vi "sqiggle_write_n.vi"(7 "I2C interface":T1, 8 "error in":errorcluster, 10 "Axis num":i32, 11 "Pulse count":i16) -> (0 "error out":errorcluster)   [LabVIEW 2013]
uses:
  i2c_interface.ctl
  fpga_reference.ctl
  Common/demux_command.ctl
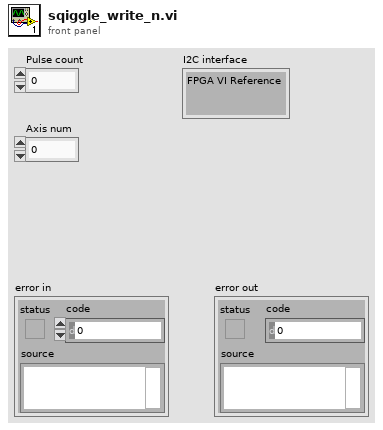
[diagram p1: front panel]
types:
  T1 = typedef "i2c_interface.ctl" = cluster{"FPGA VI Reference":T2}
  T2 = typedef "fpga_reference.ctl" = refnum<k20>
  T3 = typedef "demux_command.ctl" = enum8{"bus_0", "bus_1", "bus_2", "invalid_3", "invalid_4", "drain_fifo", "wait_hard_trigger", "wait_soft_trigger", "trigger_enable"}
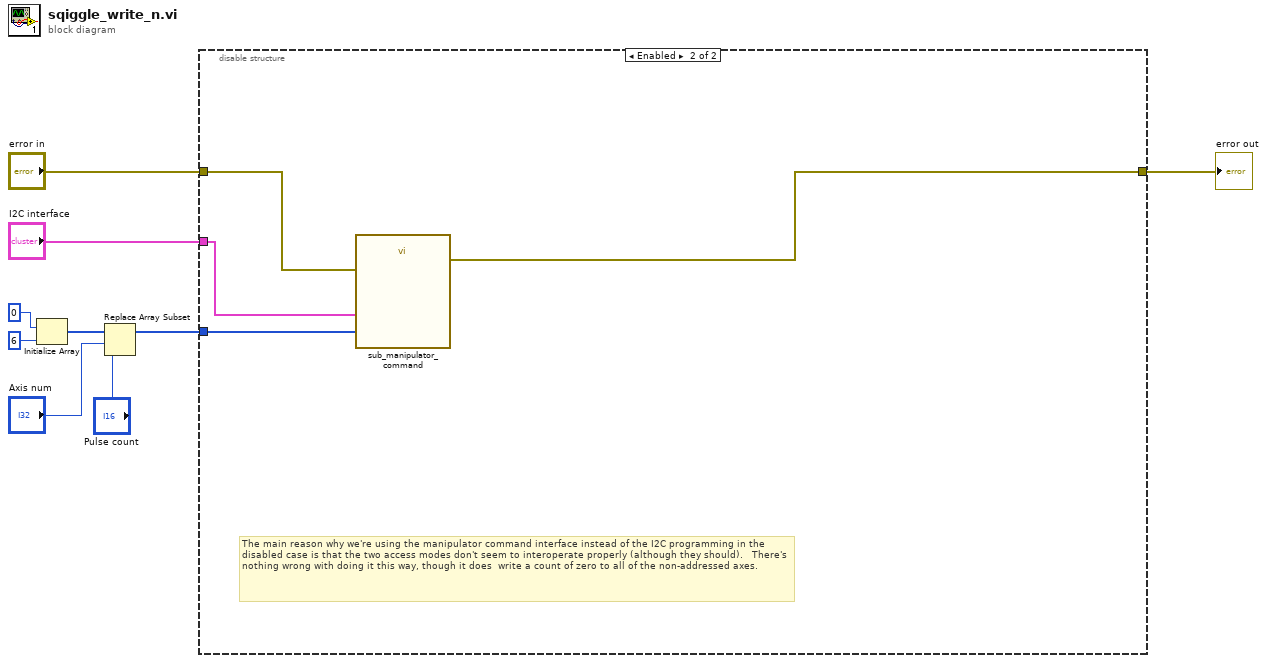
[diagram p0: block diagram]
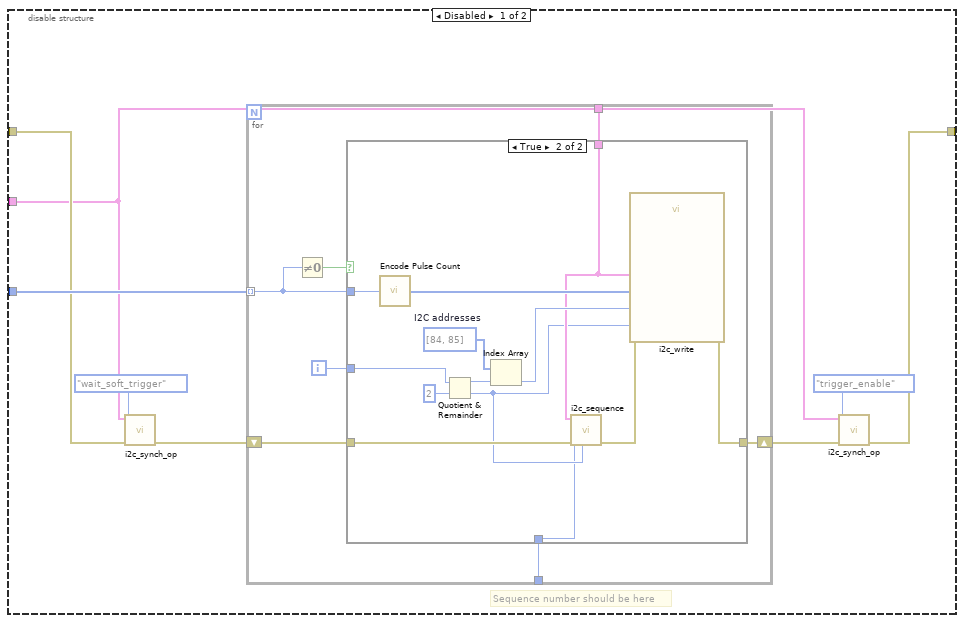
[diagram p2: hidden frame]
diagram:
  n1 = Initialize Array(i16 0 ("Pulse count"), 6 ("dimension size")) -> (w8:i16[])
  n2 = Replace Array Subset(array=w8, new element="Pulse count", index="Axis num") -> (w1:i16[])
  n3 = disable-structure shown="Enabled" {
    disable-tunnel: w1 -> [w17 w41]
    disable-tunnel: "error in" -> [w14 w40]
    disable-tunnel: [w12 w39] -> w3
    disable-tunnel: "I2C interface" -> [w11 w42]
    frame Disabled {
      # "Sequence number should be here"
      n4 = call "i2c_synch_op.vi"("error in"=w14, "Demux command"=demux_command."wait_soft_trigger", "I2C interface"=w11) -> ("error out"=w10:errorcluster)  [unwired: 7 in, 1 out]
      n5 = for {
        tunnel: w17 -> [w20] mode=indexing
        shift-right: [w23] -> w13
        shift-left: w10 -> [w24]
        tunnel: w11 -> [w21]
        tunnel: _ -> [w18]
        i -> [w22]
        n6 = Not Equal To 0?(x=w20) -> (x != 0?=w19:bool)
        n7 = case shown="True" w19 {
          tunnel: w24 -> [w25 w30]
          tunnel: [w25 w38] -> w23
          tunnel: w22 -> [_ w37]
          tunnel: w21 -> [_ w29]
          tunnel: w20 -> [_ w31]
          tunnel: w18 -> [_ w26]
          frame False {
          }
          frame True {
            w35 = u8[] [84, 85]  # I2C addresses
            n8 = call "Encode Pulse Count.vi"("Pulse count"=w31) -> ("Array"=w32:u8[])
            n9 = Quotient & Remainder(x=w37, y=2) -> (x-y*floor(x/y)=w34:i32, floor(x/y)=w28:i32)
            n10 = Index Array(array=w35, index=w34) -> (element=w33:u8)
            n11 = call "i2c_sequence.vi"("Bus"=w28, "error in"=w30, "Sequence number"=w26, "I2C interface"=w29) -> ("error out"=w27:errorcluster)  [unwired: 6 in, 1 out]
            n12 = call "i2c_write.vi"("Bus"=w28, "error in"=w27, "Data"=w32, "Address"=w33, "I2C interface"=w29) -> ("error out"=w38:errorcluster)  [unwired: 5 in, 1 out]
          }
        }
      }
      n13 = call "i2c_synch_op.vi"("error in"=w13, "Demux command"=demux_command."trigger_enable", "I2C interface"=w11) -> ("error out"=w12:errorcluster)  [unwired: 7 in, 1 out]
    }
    frame Enabled {
      # "The main reason why we're using the manipulator command interface instead of the I2C programming in the disabled case is that the two access modes don't seem to interoperate properly (although they should).   There's nothing wrong with doing it this way, though it does  write a count of zero to all of the non-addressed axes."
      n14 = call "sub_manipulator_command.vi"("error in"=w40, "Cycles"=w41, "I2C interface"=w42) -> ("error out"=w39:errorcluster)  [unwired: 8 in]
    }
  }
  "error out" <- w3
